vi "多参数 interface.vi"   [LabVIEW 2016, in "MB SLAVE.lvlib"]
uses:
  MB SLAVE.lvlib
types:
  T1 = typedef "多参数交互.ctl" = cluster{"pH":bool, "DO":bool, "Turb":bool, "Cond":bool, "Temp":bool, "叶绿素a启用":bool, "蓝绿藻":bool, "藻密度":bool, "orp":bool}
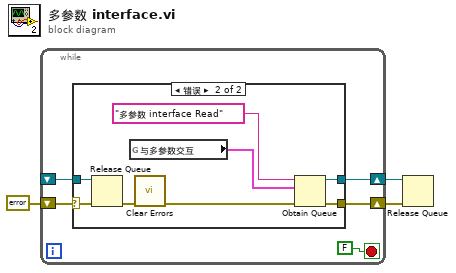
[diagram p0: block diagram]
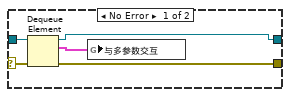
[diagram p2: hidden frame]
diagram:
  n1 = while {
    shift-right: [w8] -> w1
    shift-left: errorcluster {"status"=TRUE, "code"=0, "source"=""} ("error out") -> [w7]
    shift-right: [w6] -> w2
    shift-left: _ -> [w5]
    stop <- FALSE stop-if-true
    n2 = case shown="错误" w7 {
      selector: w7 -> [w12 w18]
      tunnel: [w10 w20] -> w8
      tunnel: [w11 w19] -> w6
      tunnel: w5 -> [w13 w17]
      frame No Error {
        n3 = Dequeue Element(queue=w13, error in (no error)=w12) -> (queue out=w11:refnum<queue>, element=w9:T1, error out=w10:errorcluster)  [unwired: 1 in, 1 out]
        n4 = global write "modbus slave全局.vi" "与多参数交互"(w9) -> ()
      }
      frame Error {
        n5 = Release Queue(queue=w17, error in (no error)=w18) -> (error out=w16:errorcluster)  [unwired: 1 in, 2 out]
        n6 = global read "modbus slave全局.vi" "与多参数交互"() -> (w14:T1)
        n7 = call <vilib>:"Clear Errors.vi"("error in (no error)"=w16) -> ("error out"=w15:errorcluster)  [unwired: 5 in, 1 out]
        n8 = Obtain Queue(name (unnamed)="多参数 interface Read" ("写入方名称"), element data type=w14, error in (no error)=w15) -> (queue out=w19:refnum<queue>, error out=w20:errorcluster)  [unwired: 2 in, 1 out]
      }
    }
  }
  n9 = Release Queue(queue=w2, error in (no error)=w1) -> ()  [unwired: 1 in, 3 out]
